vi "free_unpack.vi"(3 "error in":errorcluster, 5 "u":u64) -> (0 "error out":errorcluster)   [LabVIEW 2019, in "msgunpack.lvlib"]
doc: "Closes the msgpack object and frees any memory associated with it."
uses:
  msgunpack.lvlib
  msgpackalt.dll
panel:
  # "msgpack"
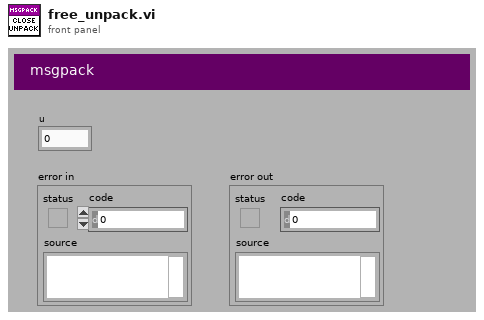
[diagram p1: front panel]
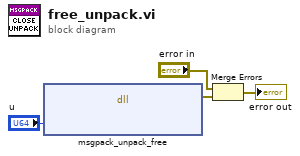
[diagram p0: block diagram]
diagram:
  n1 = dll-call lib="C:/Users/Patrick/Documents/GitHub/Instrument-Framework/lvsrc/SMOs/JSON-RPC-2019/lv-venv/lv.lib/vi.lib/addons/msgpack/msgpackalt.dll" fn="msgpack_unpack_free"("p"="u") -> (error out=w3:errorcluster)  [unwired: 5 in, 1 out]
  n2 = Merge Errors("error in", w3) -> (→"error out":errorcluster)
